vi "_loadStage.vi"(4 "error in (no error)":errorcluster, 6 "stage type":T1, 7 "_delayStageBase.lvclass":refnum<class "_delayStageBase.lvclass">) -> (0 "error out":errorcluster, 3 "_delayStageBase.lvclass":refnum<class "_delayStageBase.lvclass">)   [LabVIEW 2019, in "_delayStageBase.lvclass"]
uses:
  _delayStageBase.lvclass
  _stageType.ctl
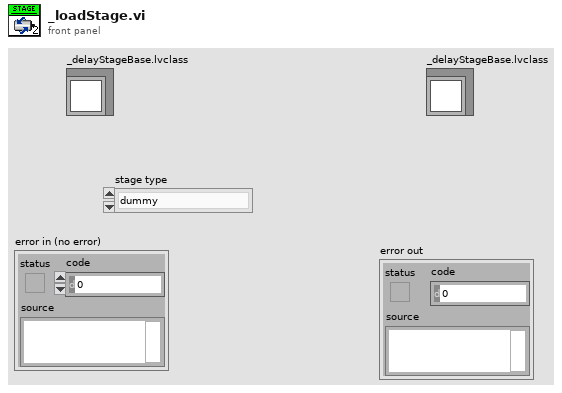
[diagram p1: front panel]
types:
  T1 = typedef "_stageType.ctl" = enum16{"dummy", "ESP300", "ESP301 via TCPIP"}
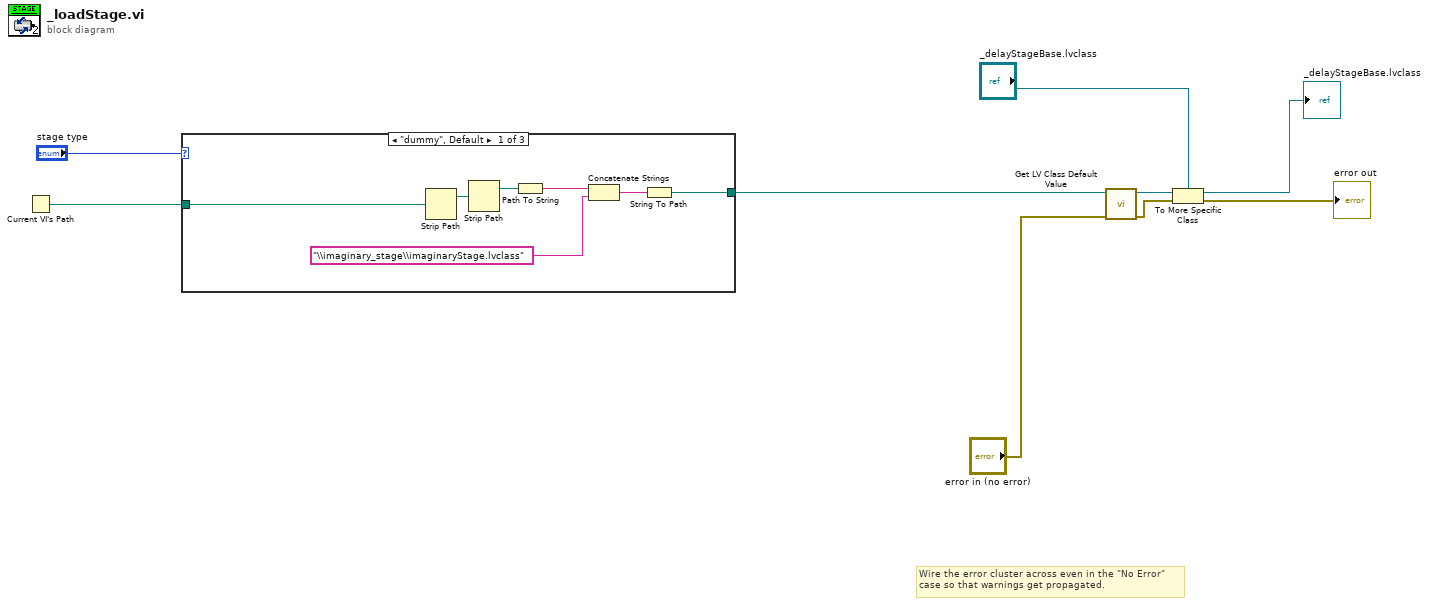
[diagram p0: block diagram]
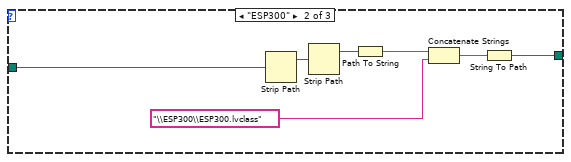
[diagram p2: hidden frame]
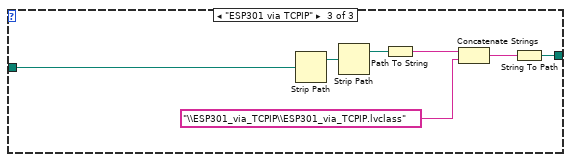
[diagram p3: hidden frame]
diagram:
  # "Wire the error cluster across even in the \"No Error\"\ncase so that warnings get propagated."
  n1 = Current VI's Path() -> (path=w3:path)
  n2 = case shown="\"dummy\", Default" "stage type" {
    tunnel: [w10 w17 w25] -> w2
    tunnel: w3 -> [w11 w18 w24]
    frame "dummy", Default {
      n3 = Strip Path(path=w11) -> (stripped path=w13:path)  [unwired: 1 out]
      n4 = Strip Path(path=w13) -> (stripped path=w14:path)  [unwired: 1 out]
      n5 = Path To String(path=w14) -> (string=w15:string)
      n6 = Concatenate Strings(w15, "\\imaginary_stage\\imaginaryStage.lvclass") -> (w16:string)
      n7 = String To Path(string=w16) -> (path=w10:path)
    }
    frame "ESP300" {
      n8 = Strip Path(path=w18) -> (stripped path=w20:path)  [unwired: 1 out]
      n9 = Strip Path(path=w20) -> (stripped path=w21:path)  [unwired: 1 out]
      n10 = Path To String(path=w21) -> (string=w22:string)
      n11 = Concatenate Strings(w22, "\\ESP300\\ESP300.lvclass") -> (w23:string)
      n12 = String To Path(string=w23) -> (path=w17:path)
    }
    frame "ESP301 via TCPIP" {
      n13 = Strip Path(path=w24) -> (stripped path=w27:path)  [unwired: 1 out]
      n14 = Strip Path(path=w27) -> (stripped path=w28:path)  [unwired: 1 out]
      n15 = Path To String(path=w28) -> (string=w29:string)
      n16 = Concatenate Strings(w29, "\\ESP301_via_TCPIP\\ESP301_via_TCPIP.lvclass") -> (w30:string)
      n17 = String To Path(string=w30) -> (path=w25:path)
    }
  }
  n18 = call <vilib>:"Get LV Class Default Value.vi"("error in (no error)"="error in (no error)", "class path"=w2) -> ("error out"=w8:errorcluster, "object"=w9:refnum<class>)  [unwired: 8 in]
  n19 = To More Specific Class(target class="_delayStageBase.lvclass", reference=w9, error in=w8) -> (specific class reference=→"_delayStageBase.lvclass":refnum<class "_delayStageBase.lvclass">, error out=→"error out":errorcluster)
